vi "convert lockin amplitude.vi"(11 "Input":i16[](array[numeric])=[0, 0]) -> (2 "x*y":dbl[](array[numeric]))   [LabVIEW 2023]
uses:
  User_Vi/Settings.vi
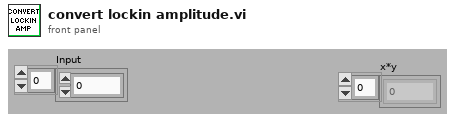
[diagram p1: front panel]
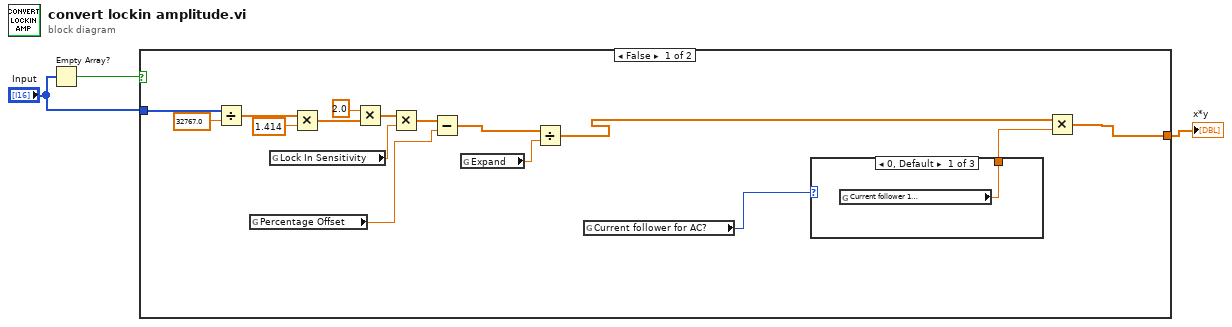
[diagram p0: block diagram]
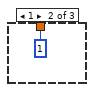
[diagram p2: hidden frame]
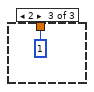
[diagram p3: hidden frame]
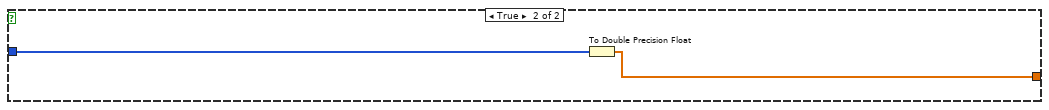
[diagram p4: hidden frame]
diagram:
  n1 = Empty Array?(array="Input") -> (empty?=w2:bool)
  n2 = case shown="False" w2 {
    tunnel: "Input" -> [w18 w24]
    tunnel: [w8 w23] -> w1
    frame False {
      n3 = Divide(x=w18, y=32767.0 ("n")) -> (x/y=w16:dbl[])
      n4 = global read "Settings.vi" "Percentage Offset"() -> (w6:dbl)
      n5 = global read "Settings.vi" "Lock In Sensitivity"() -> (w9:dbl)
      n6 = Multiply(x=w16, y=1.414) -> (x*y=w15:dbl[])
      n7 = Multiply(x=2.0 ("y"), y=w15) -> (x*y=w10:dbl[])
      n8 = Multiply(x=w10, y=w9) -> (x*y=w7:dbl[])
      n9 = Subtract(x=w7, y=w6) -> (x-y=w13:dbl[])
      n10 = global read "Settings.vi" "Expand"() -> (w12:dbl)
      n11 = Divide(x=w13, y=w12) -> (x/y=w11:dbl[])
      n12 = global read "Settings.vi" "Current follower for AC?"() -> (w4:u8)
      n13 = case shown="0, Default" w4 {
        tunnel: [w20 u16 1 ("Sensitivity") u16 1 ("Sensitivity")] -> w5
        frame 0, Default {
          n14 = global read "Settings.vi" "Current follower 1\n (AI-3)"() -> (w20:dbl)
        }
        frame 1 {
        }
        frame 2 {
        }
      }
      n15 = Multiply(x=w11, y=w5) -> (x*y=w8:dbl[])
    }
    frame True {
      n16 = To Double Precision Float(number=w24) -> (double precision float=w23:dbl[])
    }
  }
  "x*y" <- w1
